vi "Transmit.vi"(4 "Len":u32, 6 "pSend":u8[](array[numeric]), 8 "error in (no error)":errorcluster caption="错误输入（无错误）", 9 "CANInd":u32, 10 "DeviceInd":u32, 11 "type":u16(ring)=2 items=["USB-CAN"=2, "USB-CAN2.0"=3]) -> (0 "error out":errorcluster caption="错误输出", 3 "Success":u32)   [LabVIEW 2011]
uses:
  data/ControlCAN.dll
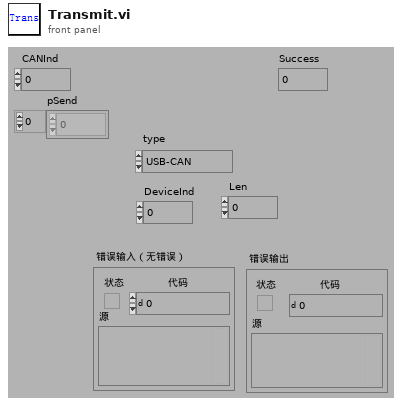
[diagram p1: front panel]
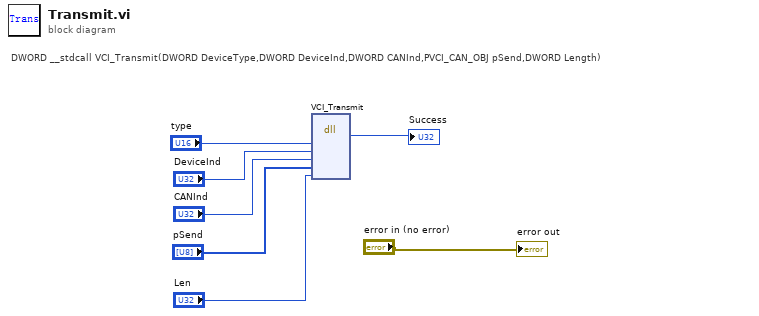
[diagram p0: block diagram]
diagram:
  # "DWORD __stdcall VCI_Transmit(DWORD DeviceType,DWORD DeviceInd,DWORD CANInd,PVCI_CAN_OBJ pSend,DWORD Length)"
  n1 = dll-call lib="PTH1vabs E工作USB-CAN Tool上位机源码USB-CAN Tool工具源码ZLG版USB CAN TooldataControlCAN.dll" fn="VCI_Transmit"("DeviceType"="type", "DeviceInd"="DeviceInd", "CANInd"="CANInd", "pSend"="pSend", "Len"="Len") -> ("返回类型"=→"Success":u32)  [unwired: 8 in, 2 out]
  "error out" <- "error in (no error)"
